vi "图像显示.vi"() -> ()   [LabVIEW 2013]
panel:
  in  "油压显示":bool
  in  "试验模式对照":dbl[](array[numeric])=[0.0, 1.0, 2.0, 3.0, 4.0, 5.0]
  in  "未做试验编号":i32[](array[numeric])
  in  "保存图像":bool
  out "两条曲线":cluster{dbl, "Sampling Rate":dbl, dbl[][]}(graph) caption="油压"
  in  "试验模式":u16(ring) items=["快关L1L2", "快关L1", "快关L2", "步响应1", "归零", "开启关闭", "油压"]
  in  "stop":bool
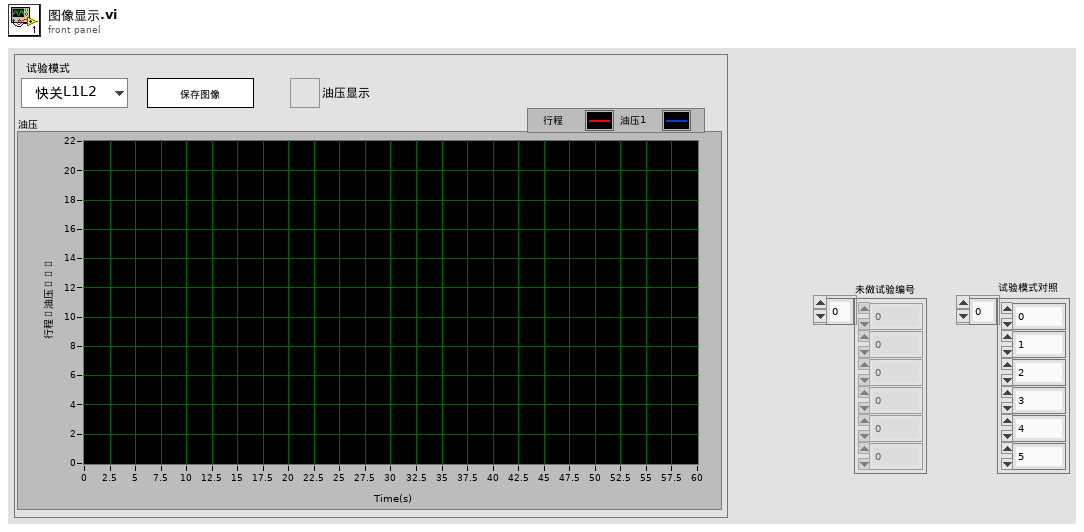
[diagram p1: front panel]
types:
  T1 = cluster{"tv1":dbl, "tv2":dbl, "tv":dbl, "ts1":dbl, "ts2":dbl, "ts":dbl, "td1":dbl, "td":dbl, "Slope":dbl, "Intercept":dbl, "I100":dbl, "I0":dbl, "Sen":dbl, "V1":dbl, "V2":dbl, "CL":dbl, "OP":dbl, "DFT":dbl}
  T2 = cluster{"X_value_start":dbl, "X_value_peak":dbl, "t1":dbl, "X_value_end":dbl, "V0":dbl, "V1":dbl, "t0":dbl, "X_peaks":dbl[], "X_valleys":dbl[], "Y_peaks":dbl[], "Y_valleys":dbl[], "t2":dbl, "H_overshoot":dbl, "T_overshoot":dbl, "T_entitre_overshoot":dbl, "X_value_start 2":dbl, "X_value_peak 2":dbl, "t1 2":dbl, "X_value_end 2":dbl, "V0 2":dbl, "V1 2":dbl, "t0 2":dbl, "X_peaks 2":dbl[], "X_valleys 2":dbl[], "Y_peaks 2":dbl[], "t2 2":dbl, "H_overshoot 2":dbl, "T_overshoot 2":dbl, "T_entitre_overshoot 2":dbl, "Y_valleys 2":dbl[]}
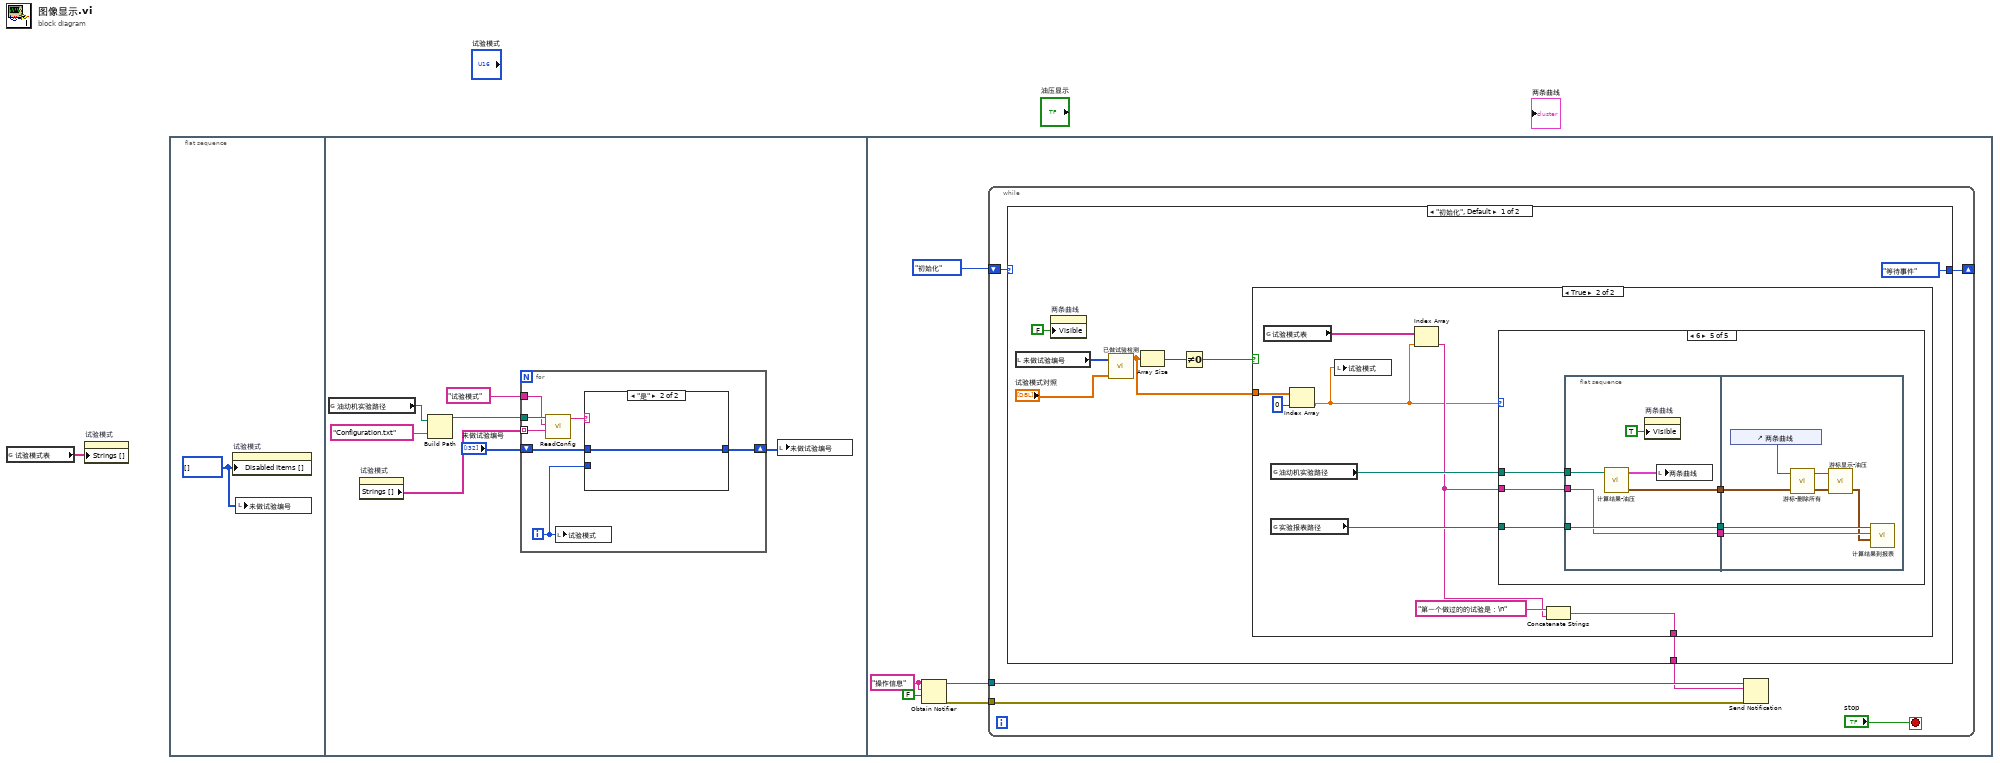
[diagram p0: block diagram]
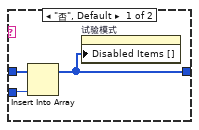
[diagram p2: hidden frame]
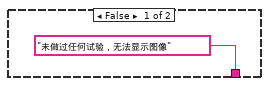
[diagram p3: hidden frame]
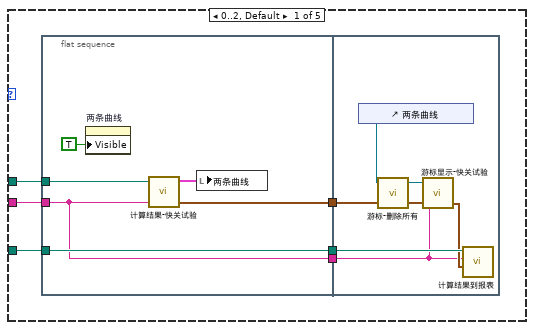
[diagram p4: hidden frame]
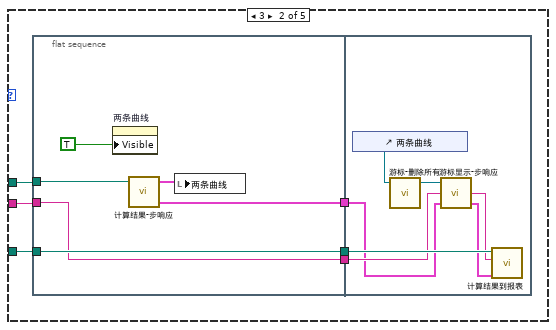
[diagram p5: hidden frame]
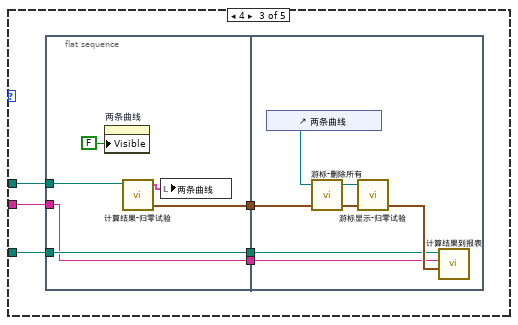
[diagram p6: hidden frame]
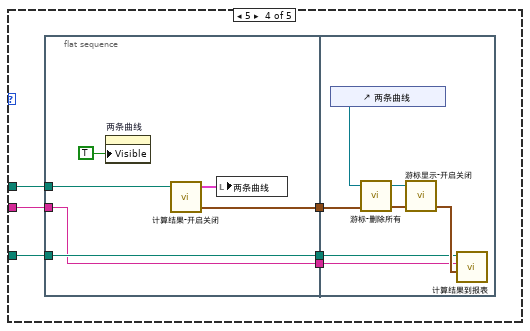
[diagram p7: hidden frame]
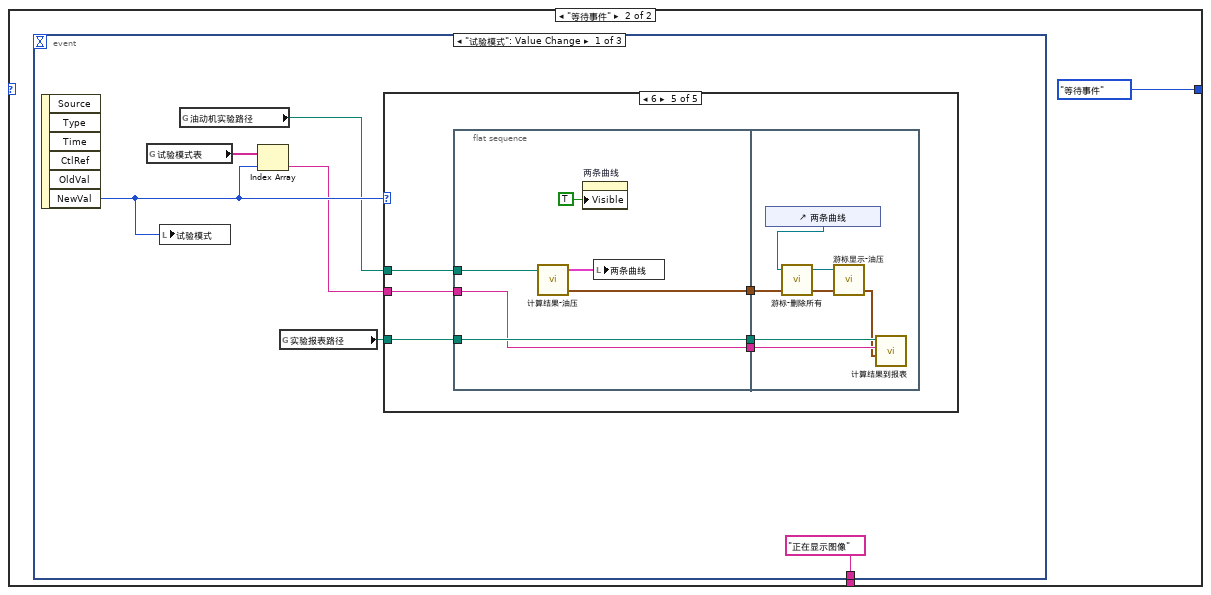
[diagram p8: hidden frame]
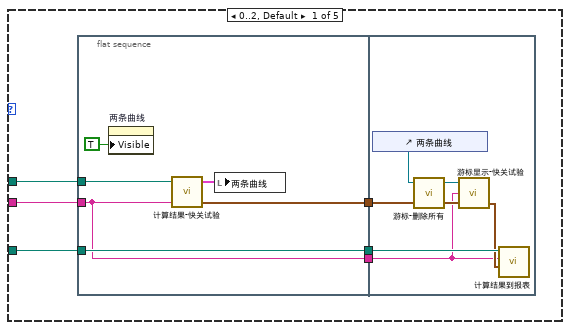
[diagram p9: hidden frame]
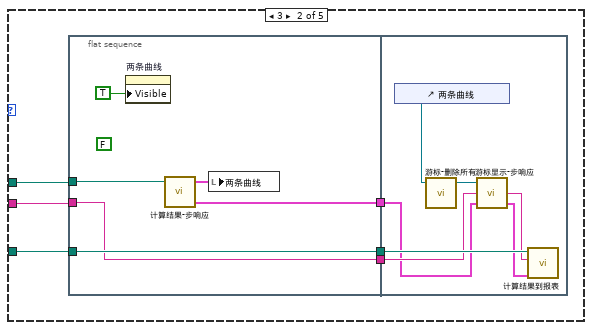
[diagram p10: hidden frame]
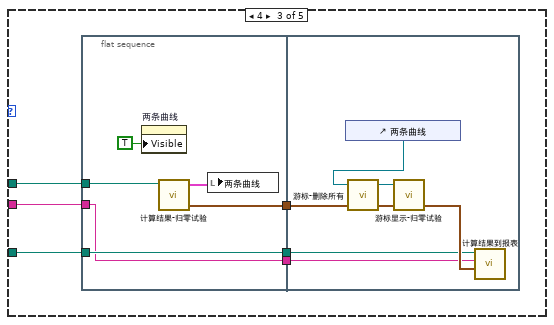
[diagram p11: hidden frame]
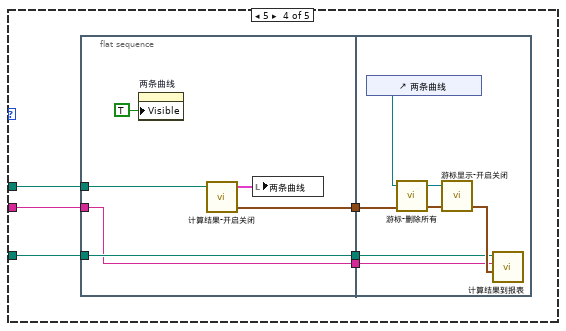
[diagram p12: hidden frame]
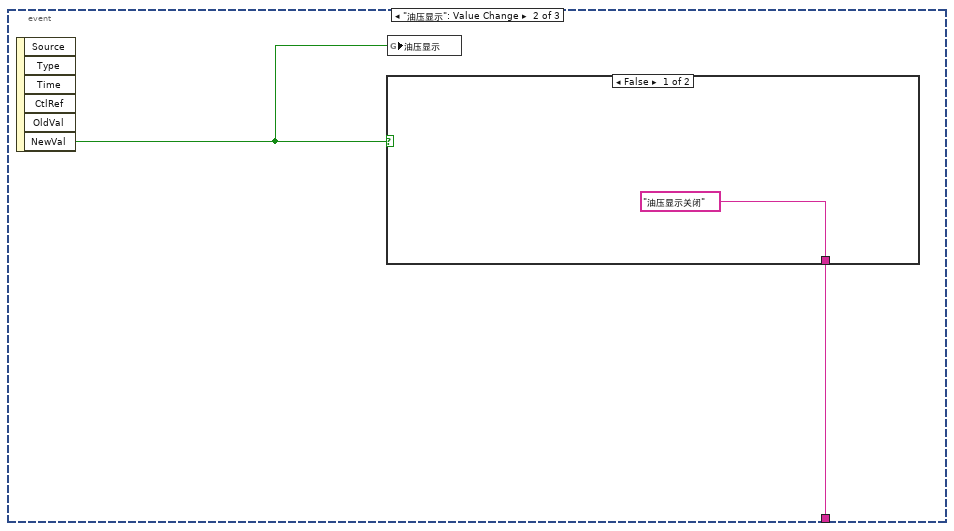
[diagram p13: hidden frame]
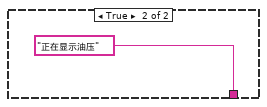
[diagram p14: hidden frame]
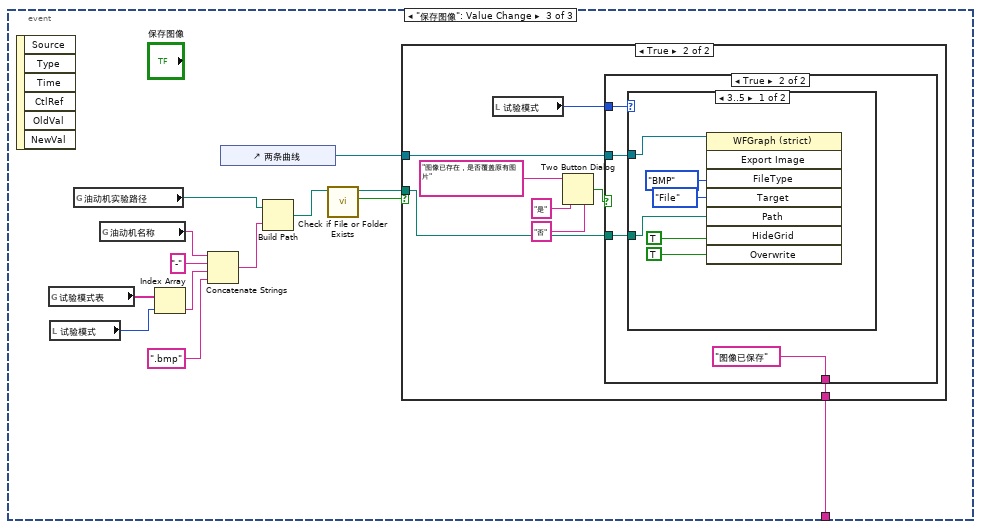
[diagram p15: hidden frame]
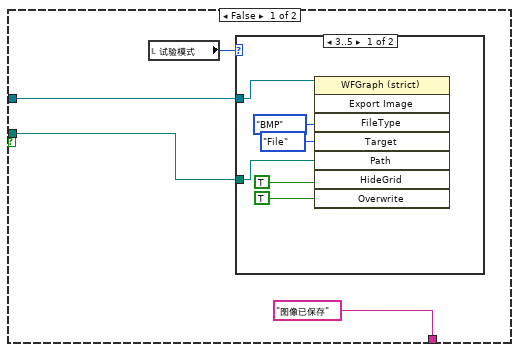
[diagram p16: hidden frame]
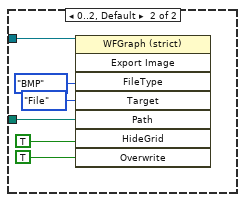
[diagram p17: hidden frame]
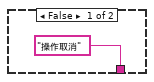
[diagram p18: hidden frame]
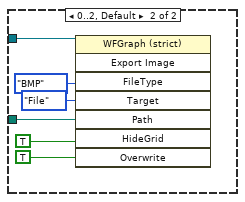
[diagram p19: hidden frame]
diagram:
  n1 = global read "试验模式表.vi" "试验模式表"() -> (w1:string[])
  n2 = property on="试验模式" class="Ring (strict)"("Strings []"=w1) -> ()  [unwired: 2 in, 2 out]
  n3 = flat-sequence {
    frame #0 {
      w2 = i32[] [] ("Disabled Items []")
      n4 = property on="试验模式" class="Ring (strict)"("Disabled Items []"=w2) -> ()  [unwired: 2 in, 2 out]
      n5 = local write "未做试验编号"(w2) -> ()
    }
    frame #1 {
      n6 = global read "油动机实验路径.vi" "油动机实验路径"() -> (w8:path)
      n7 = property on="试验模式" class="Ring (strict)"() -> ("Strings []"=w6:string[])  [unwired: 2 in, 2 out]
      n8 = Build Path(base path=w8, name or relative path="Configuration.txt" ("名称或相对路径")) -> (appended path=w7:path)
      n9 = for {
        tunnel: w7 -> [w16]
        tunnel: w6 -> [w15] mode=indexing
        tunnel: "试验模式" -> [w14]
        shift-right: [w11] -> w3
        shift-left: "未做试验编号" -> [w10]
        i -> [w12]
        n10 = call "ReadConfig.vi"("Key"=w15, "Section"=w14, "Path"=w16) -> ("Value"=w13:string)  [unwired: 1 in, 2 out]
        n11 = local write "试验模式"(w12) -> ()
        n12 = case shown="\"是\"" w13 {
          tunnel: w12 -> [w19 _]
          tunnel: [w18 w20] -> w11
          tunnel: w10 -> [w17 w20]
          frame "否", Default {
            n13 = Insert Into Array(array=w17, new element=w19) -> (w18:i32[])  [unwired: 1 in]
            n14 = property on="试验模式" class="Ring (strict)"("Disabled Items []"=w18) -> ()  [unwired: 2 in, 2 out]
          }
          frame "是" {
          }
        }
      }
      n15 = local write "未做试验编号"(w3) -> ()
    }
    frame #2 {
      w24 = "操作信息" ("name (unnamed)")
      n16 = Obtain Notifier(name (unnamed)=w24, notification data type=w24, create if not found? (T)=FALSE) -> (notifier out=w23:refnum<notifier>, error out=w22:errorcluster)  [unwired: 1 in, 1 out]
      n17 = while {
        shift-right: [w29] -> _
        shift-left: enum16{"初始化", "等待事件"}."初始化" -> [w30]
        tunnel: w23 -> [w28]
        tunnel: w22 -> [w27]
        stop <- "stop" stop-if-true
        n18 = case shown="\"初始化\", Default" w30 {
          tunnel: [enum16{"初始化", "等待事件"}."等待事件" enum16{"初始化", "等待事件"}."等待事件"] -> w29
          tunnel: [w37 w141] -> w26
          frame "初始化", Default {
            n19 = local read "未做试验编号"() -> (w35:i32[])
            n20 = property on="两条曲线" class="WFGraph (strict)"("Visible"=FALSE) -> ()  [unwired: 2 in, 2 out]
            n21 = call "已做试验检测.vi"("试验模式编号"="试验模式对照", "未做试验编号"=w35) -> ("已做试验编号"=w32:dbl[])  [unwired: 3 in]
            n22 = Array Size(array=w32) -> (size(s)=w34:i32)
            n23 = Not Equal To 0?(x=w34) -> (x != 0?=w33:bool)
            n24 = case shown="True" w33 {
              tunnel: ["未做过任何试验，无法显示图像" w44] -> w37
              tunnel: w32 -> [_ w42]
              frame False {
              }
              frame True {
                n25 = global read "试验模式表.vi" "试验模式表"() -> (w49:string[])
                n26 = global read "油动机实验路径.vi" "油动机实验路径"() -> (w48:path)
                n27 = global read "实验报表路径.vi" "实验报表路径"() -> (w47:path)
                n28 = Index Array(array=w42, index=0) -> (element=w41:dbl)
                n29 = local write "试验模式"(w41) -> ()
                n30 = Index Array(array=w49, index=w41) -> (element=w45:string)
                n31 = case shown="6" w41 {
                  tunnel: w48 -> [w55 w69 w92 w110 w128]
                  tunnel: w45 -> [w53 w70 w87 w105 w123]
                  tunnel: w47 -> [w54 w71 w89 w108 w125]
                  frame 0..2, Default {
                    n32 = flat-sequence {
                      tunnel: w55 -> [w61]
                      tunnel: w54 -> [w59]
                      tunnel: w53 -> [w58]
                      tunnel: [w60] -> w52
                      tunnel: [w59] -> w51
                      tunnel: [w58] -> w50
                      tunnel: w52 -> [w66]
                      tunnel: w51 -> [w65]
                      tunnel: w50 -> [w63]
                      frame #0 {
                        n33 = property on="两条曲线" class="WFGraph (strict)"("Visible"=TRUE) -> ()  [unwired: 2 in, 2 out]
                        n34 = call "计算结果-快关试验.vi"("试验模式"=w58, "油动机试验路径"=w61) -> ("计算参数 out"=w60:T1, "快关实验"=w56:cluster{dbl, "Sampling Rate":dbl, dbl[][]})  [unwired: 1 in, 1 out]
                        n35 = local write "两条曲线"(w56) -> ()
                      }
                      frame #1 {
                        n36 = control-ref of="两条曲线"() -> (w62:refnum<vi>)
                        n37 = call "游标-删除所有.vi"("reference in"=w62) -> ("reference out"=w67:refnum<vi>)  [unwired: 4 in]
                        n38 = call "游标显示-快关试验.vi"("计算参数 in"=w66, "试验模式"=w63, "reference in"=w67) -> ("计算参数 out"=w64:T1)  [unwired: 1 in, 1 out]
                        n39 = call "计算结果到报表.vi"("计算参数"=w64, "试验模式"=w63, "试验报表路径"=w65) -> ()  [unwired: 1 in]
                      }
                    }
                  }
                  frame 3 {
                    n40 = flat-sequence {
                      tunnel: w69 -> [w77]
                      tunnel: w71 -> [w79]
                      tunnel: w70 -> [w78]
                      tunnel: [w79] -> w73
                      tunnel: [w78] -> w72
                      tunnel: [w76] -> w68
                      tunnel: w73 -> [w86]
                      tunnel: w72 -> [w84]
                      tunnel: w68 -> [w83]
                      frame #0 {
                        n41 = property on="两条曲线" class="WFGraph (strict)"("Visible"=TRUE) -> ()  [unwired: 2 in, 2 out]
                        n42 = call "计算结果-步响应.vi"("油动机试验路径"=w77) -> ("步响应计算参数 out"=w76:T2, "波形图"=w74:cluster{dbl, dbl, dbl[][]})  [unwired: 3 in]
                        n43 = local write "两条曲线"(w74) -> ()
                      }
                      frame #1 {
                        n44 = control-ref of="两条曲线"() -> (w80:refnum<vi>)
                        n45 = call "游标-删除所有.vi"("reference in"=w80) -> ("reference out"=w85:refnum<vi>)  [unwired: 4 in]
                        n46 = call "游标显示-步响应.vi"("步响应计算参数 in"=w83, "试验模式"=w84, "reference in"=w85) -> ("步响应计算参数 out"=w82:T2, "试验模式 out"=w81:string)  [unwired: 1 out]
                        n47 = call "计算结果到报表.vi"("步响应计算参数"=w82, "试验模式"=w81, "试验报表路径"=w86) -> ()  [unwired: 1 in]
                      }
                    }
                  }
                  frame 4 {
                    n48 = flat-sequence {
                      tunnel: w92 -> [w98]
                      tunnel: [w97] -> w91
                      tunnel: [w96] -> w90
                      tunnel: w89 -> [w96]
                      tunnel: [w95] -> w88
                      tunnel: w87 -> [w95]
                      tunnel: w91 -> [w102]
                      tunnel: w90 -> [w101]
                      tunnel: w88 -> [w100]
                      frame #0 {
                        n49 = property on="两条曲线" class="WFGraph (strict)"("Visible"=FALSE) -> ()  [unwired: 2 in, 2 out]
                        n50 = call "计算结果-归零试验.vi"("油动机试验路径"=w98) -> ("计算参数 out"=w97:T1, "波形图"=w93:cluster{dbl, dbl, dbl[][]})  [unwired: 2 in, 1 out]
                        n51 = local write "两条曲线"(w93) -> ()
                      }
                      frame #1 {
                        n52 = control-ref of="两条曲线"() -> (w99:refnum<vi>)
                        n53 = call "游标-删除所有.vi"("reference in"=w99) -> ("reference out"=w103:refnum<vi>)  [unwired: 4 in]
                        n54 = call "游标显示-归零试验.vi"("计算参数 in"=w102, "reference in"=w103) -> ("计算参数 out"=w104:T1)  [unwired: 2 in, 1 out]
                        n55 = call "计算结果到报表.vi"("计算参数"=w104, "试验模式"=w100, "试验报表路径"=w101) -> ()  [unwired: 1 in]
                      }
                    }
                  }
                  frame 5 {
                    n56 = flat-sequence {
                      tunnel: w110 -> [w116]
                      tunnel: [w114] -> w109
                      tunnel: w108 -> [w113]
                      tunnel: [w113] -> w107
                      tunnel: [w112] -> w106
                      tunnel: w105 -> [w112]
                      tunnel: w109 -> [w120]
                      tunnel: w107 -> [w119]
                      tunnel: w106 -> [w118]
                      frame #0 {
                        n57 = property on="两条曲线" class="WFGraph (strict)"("Visible"=TRUE) -> ()  [unwired: 2 in, 2 out]
                        n58 = call "计算结果-开启关闭.vi"("油动机试验路径"=w116) -> ("计算参数 out"=w114:T1, "开启关闭试验"=w115:cluster{dbl, dbl, dbl[][]})  [unwired: 2 in, 1 out]
                        n59 = local write "两条曲线"(w115) -> ()
                      }
                      frame #1 {
                        n60 = control-ref of="两条曲线"() -> (w117:refnum<vi>)
                        n61 = call "游标-删除所有.vi"("reference in"=w117) -> ("reference out"=w121:refnum<vi>)  [unwired: 4 in]
                        n62 = call "游标显示-开启关闭.vi"("计算参数 in"=w120, "reference in"=w121) -> ("计算参数 out"=w122:T1)  [unwired: 2 in, 1 out]
                        n63 = call "计算结果到报表.vi"("计算参数"=w122, "试验模式"=w118, "试验报表路径"=w119) -> ()  [unwired: 1 in]
                      }
                    }
                  }
                  frame 6 {
                    n64 = flat-sequence {
                      tunnel: w128 -> [w134]
                      tunnel: [w132] -> w127
                      tunnel: [w131] -> w126
                      tunnel: w125 -> [w131]
                      tunnel: [w130] -> w124
                      tunnel: w123 -> [w130]
                      tunnel: w127 -> [w140]
                      tunnel: w126 -> [w137]
                      tunnel: w124 -> [w136]
                      frame #0 {
                        n65 = call "计算结果-油压.vi"("油动机试验路径"=w134) -> ("计算参数 out"=w132:T1, "油压"=w133:cluster{dbl, dbl, dbl[][]})  [unwired: 2 in, 1 out]
                        n66 = property on="两条曲线" class="WFGraph (strict)"("Visible"=TRUE) -> ()  [unwired: 2 in, 2 out]
                        n67 = local write "两条曲线"(w133) -> ()
                      }
                      frame #1 {
                        n68 = control-ref of="两条曲线"() -> (w138:refnum<vi>)
                        n69 = call "游标-删除所有.vi"("reference in"=w138) -> ("reference out"=w139:refnum<vi>)  [unwired: 4 in]
                        n70 = call "游标显示-油压.vi"("计算参数 in"=w140, "reference in"=w139) -> ("计算参数 out"=w135:T1)  [unwired: 2 in, 1 out]
                        n71 = call "计算结果到报表.vi"("计算参数"=w135, "试验模式"=w136, "试验报表路径"=w137) -> ()  [unwired: 1 in]
                      }
                    }
                  }
                }
                n72 = Concatenate Strings("第一个做过的的试验是：\n", w45) -> (w44:string)
              }
            }
          }
          frame "等待事件" {
            n73 = event shown="[0] \"试验模式\": Value Change" {
              selector: _ -> [_ _ _]
              dyn-events: _ -> [_ _ _]
              timeout: _ -> [_ _ _]
              tunnel: ["正在显示图像" w240 w244] -> w141
              event "试验模式": Value Change {
                n74 = event-data() -> ("NewVal"=w146:u16)  [unwired: 1 in, 5 out]
                n75 = global read "试验模式表.vi" "试验模式表"() -> (w148:string[])
                n76 = local write "试验模式"(w146) -> ()
                n77 = global read "油动机实验路径.vi" "油动机实验路径"() -> (w145:path)
                n78 = Index Array(array=w148, index=w146) -> (element=w144:string)
                n79 = global read "实验报表路径.vi" "实验报表路径"() -> (w143:path)
                n80 = case shown="6" w146 {
                  tunnel: w145 -> [w154 w168 w191 w209 w227]
                  tunnel: w144 -> [w152 w169 w186 w204 w223]
                  tunnel: w143 -> [w153 w170 w188 w207 w225]
                  frame 0..2, Default {
                    n81 = flat-sequence {
                      tunnel: w154 -> [w160]
                      tunnel: w153 -> [w156]
                      tunnel: w152 -> [w155]
                      tunnel: [w157] -> w151
                      tunnel: [w156] -> w150
                      tunnel: [w155] -> w149
                      tunnel: w151 -> [w164]
                      tunnel: w150 -> [w163]
                      tunnel: w149 -> [w161]
                      frame #0 {
                        n82 = property on="两条曲线" class="WFGraph (strict)"("Visible"=TRUE) -> ()  [unwired: 2 in, 2 out]
                        n83 = call "计算结果-快关试验.vi"("试验模式"=w155, "油动机试验路径"=w160) -> ("计算参数 out"=w157:T1, "快关实验"=w158:cluster{dbl, "Sampling Rate":dbl, dbl[][]})  [unwired: 1 in, 1 out]
                        n84 = local write "两条曲线"(w158) -> ()
                      }
                      frame #1 {
                        n85 = control-ref of="两条曲线"() -> (w166:refnum<vi>)
                        n86 = call "游标-删除所有.vi"("reference in"=w166) -> ("reference out"=w165:refnum<vi>)  [unwired: 4 in]
                        n87 = call "游标显示-快关试验.vi"("计算参数 in"=w164, "试验模式"=w161, "reference in"=w165) -> ("计算参数 out"=w162:T1)  [unwired: 1 in, 1 out]
                        n88 = call "计算结果到报表.vi"("计算参数"=w162, "试验模式"=w161, "试验报表路径"=w163) -> ()  [unwired: 1 in]
                      }
                    }
                  }
                  frame 3 {
                    n89 = flat-sequence {
                      tunnel: w168 -> [w176]
                      tunnel: w170 -> [w178]
                      tunnel: w169 -> [w177]
                      tunnel: [w178] -> w172
                      tunnel: [w177] -> w171
                      tunnel: [w174] -> w167
                      tunnel: w172 -> [w185]
                      tunnel: w171 -> [w183]
                      tunnel: w167 -> [w182]
                      frame #0 {
                        (unwired) FALSE ("Visible")
                        n90 = property on="两条曲线" class="WFGraph (strict)"("Visible"=TRUE) -> ()  [unwired: 2 in, 2 out]
                        n91 = call "计算结果-步响应.vi"("油动机试验路径"=w176) -> ("步响应计算参数 out"=w174:T2, "波形图"=w173:cluster{dbl, dbl, dbl[][]})  [unwired: 3 in]
                        n92 = local write "两条曲线"(w173) -> ()
                      }
                      frame #1 {
                        n93 = control-ref of="两条曲线"() -> (w179:refnum<vi>)
                        n94 = call "游标-删除所有.vi"("reference in"=w179) -> ("reference out"=w184:refnum<vi>)  [unwired: 4 in]
                        n95 = call "游标显示-步响应.vi"("步响应计算参数 in"=w182, "试验模式"=w183, "reference in"=w184) -> ("步响应计算参数 out"=w181:T2, "试验模式 out"=w180:string)  [unwired: 1 out]
                        n96 = call "计算结果到报表.vi"("步响应计算参数"=w181, "试验模式"=w180, "试验报表路径"=w185) -> ()  [unwired: 1 in]
                      }
                    }
                  }
                  frame 4 {
                    n97 = flat-sequence {
                      tunnel: w191 -> [w197]
                      tunnel: [w195] -> w190
                      tunnel: [w194] -> w189
                      tunnel: w188 -> [w194]
                      tunnel: [w193] -> w187
                      tunnel: w186 -> [w193]
                      tunnel: w190 -> [w201]
                      tunnel: w189 -> [w200]
                      tunnel: w187 -> [w199]
                      frame #0 {
                        n98 = property on="两条曲线" class="WFGraph (strict)"("Visible"=TRUE) -> ()  [unwired: 2 in, 2 out]
                        n99 = call "计算结果-归零试验.vi"("油动机试验路径"=w197) -> ("计算参数 out"=w195:T1, "波形图"=w192:cluster{dbl, dbl, dbl[][]})  [unwired: 2 in, 1 out]
                        n100 = local write "两条曲线"(w192) -> ()
                      }
                      frame #1 {
                        n101 = control-ref of="两条曲线"() -> (w198:refnum<vi>)
                        n102 = call "游标-删除所有.vi"("reference in"=w198) -> ("reference out"=w202:refnum<vi>)  [unwired: 4 in]
                        n103 = call "游标显示-归零试验.vi"("计算参数 in"=w201, "reference in"=w202) -> ("计算参数 out"=w203:T1)  [unwired: 2 in, 1 out]
                        n104 = call "计算结果到报表.vi"("计算参数"=w203, "试验模式"=w199, "试验报表路径"=w200) -> ()  [unwired: 1 in]
                      }
                    }
                  }
                  frame 5 {
                    n105 = flat-sequence {
                      tunnel: w209 -> [w214]
                      tunnel: [w212] -> w208
                      tunnel: w207 -> [w211]
                      tunnel: [w211] -> w206
                      tunnel: [w210] -> w205
                      tunnel: w204 -> [w210]
                      tunnel: w208 -> [w218]
                      tunnel: w206 -> [w217]
                      tunnel: w205 -> [w216]
                      frame #0 {
                        n106 = property on="两条曲线" class="WFGraph (strict)"("Visible"=TRUE) -> ()  [unwired: 2 in, 2 out]
                        n107 = call "计算结果-开启关闭.vi"("油动机试验路径"=w214) -> ("计算参数 out"=w212:T1, "开启关闭试验"=w213:cluster{dbl, dbl, dbl[][]})  [unwired: 2 in, 1 out]
                        n108 = local write "两条曲线"(w213) -> ()
                      }
                      frame #1 {
                        n109 = control-ref of="两条曲线"() -> (w221:refnum<vi>)
                        n110 = call "游标-删除所有.vi"("reference in"=w221) -> ("reference out"=w219:refnum<vi>)  [unwired: 4 in]
                        n111 = call "游标显示-开启关闭.vi"("计算参数 in"=w218, "reference in"=w219) -> ("计算参数 out"=w220:T1)  [unwired: 2 in, 1 out]
                        n112 = call "计算结果到报表.vi"("计算参数"=w220, "试验模式"=w216, "试验报表路径"=w217) -> ()  [unwired: 1 in]
                      }
                    }
                  }
                  frame 6 {
                    n113 = flat-sequence {
                      tunnel: w227 -> [w233]
                      tunnel: [w231] -> w226
                      tunnel: w225 -> [w231]
                      tunnel: [w230] -> w224
                      tunnel: w223 -> [w230]
                      tunnel: [w228] -> w222
                      tunnel: w226 -> [w237]
                      tunnel: w224 -> [w236]
                      tunnel: w222 -> [w234]
                      frame #0 {
                        n114 = call "计算结果-油压.vi"("油动机试验路径"=w233) -> ("计算参数 out"=w228:T1, "油压"=w232:cluster{dbl, dbl, dbl[][]})  [unwired: 2 in, 1 out]
                        n115 = property on="两条曲线" class="WFGraph (strict)"("Visible"=TRUE) -> ()  [unwired: 2 in, 2 out]
                        n116 = local write "两条曲线"(w232) -> ()
                      }
                      frame #1 {
                        n117 = control-ref of="两条曲线"() -> (w239:refnum<vi>)
                        n118 = call "游标-删除所有.vi"("reference in"=w239) -> ("reference out"=w238:refnum<vi>)  [unwired: 4 in]
                        n119 = call "游标显示-油压.vi"("计算参数 in"=w234, "reference in"=w238) -> ("计算参数 out"=w235:T1)  [unwired: 2 in, 1 out]
                        n120 = call "计算结果到报表.vi"("计算参数"=w235, "试验模式"=w236, "试验报表路径"=w237) -> ()  [unwired: 1 in]
                      }
                    }
                  }
                }
              }
              event "油压显示": Value Change {
                n121 = event-data() -> ("NewVal"=w241:bool)  [unwired: 1 in, 5 out]
                n122 = case shown="False" w241 {
                  tunnel: ["油压显示关闭" "正在显示油压"] -> w240
                  frame False {
                  }
                  frame True {
                  }
                }
                n123 = global write "油压显示.vi" "油压显示"(w241) -> ()
              }
              event "保存图像": Value Change {
                n124 = event-data() -> ()  [unwired: 1 in, 6 out]
                n125 = global read "试验模式表.vi" "试验模式表"() -> (w254:string[])
                n126 = local read "试验模式"() -> (w253:u16)
                n127 = global read "油动机实验路径.vi" "油动机实验路径"() -> (w248:path)
                n128 = global read "油动机名称.vi" "油动机名称"() -> (w252:string)
                n129 = Index Array(array=w254, index=w253) -> (element=w250:string)
                n130 = Concatenate Strings(w252, "-", w250, ".bmp") -> (w247:string)
                n131 = control-ref of="两条曲线"() -> (w255:refnum<vi>)
                n132 = Build Path(base path=w248, name or relative path=w247) -> (appended path=w246:path)
                n133 = call <vilib>:"Check if File or Folder Exists.vi"("path"=w246) -> ("file or folder exists?"=w256:bool, "dup path"=w245:path)  [unwired: 8 in, 1 out]
                n134 = case shown="True" w256 {
                  tunnel: w255 -> [w260 w280]
                  tunnel: w245 -> [w259 w274]
                  tunnel: ["图像已保存" w273] -> w244
                  frame False {
                    n135 = local read "试验模式"() -> (w258:u16)
                    n136 = case shown="3..5" w258 {
                      tunnel: w260 -> [w261 w269]
                      tunnel: w259 -> [w262 w267]
                      frame 3..5 {
                        n137 = invoke on="Invoke Node" class="WFGraph (strict)" method="Export Image"(reference=w261, "FileType"=enum32{"BMP", "EPS", "EMF", "PICT"}."BMP" ("文件类型"), "Target"=enum32{"File", "Clipboard"}."File", "Path"=w262, "HideGrid"=TRUE ("始终覆盖"), "Overwrite"=TRUE ("始终覆盖")) -> ()  [unwired: 2 in, 8 out]
                      }
                      frame 0..2, Default {
                        n138 = invoke on="Invoke Node" class="WFGraph (strict)" method="Export Image"(reference=w269, "FileType"=enum32{"BMP", "EPS", "EMF", "PICT"}."BMP" ("文件类型"), "Target"=enum32{"File", "Clipboard"}."File", "Path"=w267, "HideGrid"=TRUE ("始终覆盖"), "Overwrite"=TRUE ("始终覆盖")) -> ()  [unwired: 2 in, 8 out]
                      }
                    }
                  }
                  frame True {
                    n139 = local read "试验模式"() -> (w276:u16)
                    n140 = Two Button Dialog(message="图像已存在，是否覆盖原有图片", 1:"否" ("F button name (\"Cancel\")"), 2:"是" ("T button name (\"OK\")")) -> (T button?=w275:bool)
                    n141 = case shown="True" w275 {
                      tunnel: w280 -> [_ w285]
                      tunnel: w276 -> [_ w284]
                      tunnel: w274 -> [_ w283]
                      tunnel: ["操作取消" "图像已保存"] -> w273
                      frame False {
                      }
                      frame True {
                        n142 = case shown="3..5" w284 {
                          tunnel: w285 -> [w286 w294]
                          tunnel: w283 -> [w287 w292]
                          frame 3..5 {
                            n143 = invoke on="Invoke Node" class="WFGraph (strict)" method="Export Image"(reference=w286, "FileType"=enum32{"BMP", "EPS", "EMF", "PICT"}."BMP" ("文件类型"), "Target"=enum32{"File", "Clipboard"}."File", "Path"=w287, "HideGrid"=TRUE ("始终覆盖"), "Overwrite"=TRUE ("始终覆盖")) -> ()  [unwired: 2 in, 8 out]
                          }
                          frame 0..2, Default {
                            n144 = invoke on="Invoke Node" class="WFGraph (strict)" method="Export Image"(reference=w294, "FileType"=enum32{"BMP", "EPS", "EMF", "PICT"}."BMP" ("文件类型"), "Target"=enum32{"File", "Clipboard"}."File", "Path"=w292, "HideGrid"=TRUE ("始终覆盖"), "Overwrite"=TRUE ("始终覆盖")) -> ()  [unwired: 2 in, 8 out]
                          }
                        }
                      }
                    }
                  }
                }
              }
            }
          }
        }
        n145 = Send Notification(notification=w26, notifier=w28, error in (no error)=w27) -> ()  [unwired: 2 out]
      }
    }
  }
